vi "DidStop.vi"(6 "Wait for Module to stop?":bool, 7 "Exit via Stop Module Req?":bool, 8 "error in (no error)":errorcluster, 11 "ModuleAdmin":refnum<class "ModuleAdmin.lvclass">) -> (0 "error out":errorcluster, 3 "ModuleAdmin":refnum<class "ModuleAdmin.lvclass">)   [LabVIEW 2018, in "AcPwrPlugins.lvlib"]
doc: "This VI sends a stop message via a user event to Main.vi."
uses:
  AcPwrPlugins.lvlib
  <userlib>/NIST/ModuleAdminLib/ModuleAdmin/ModuleAdmin.lvclass
  AcPwrShared/clStopArgument.ctl
  AcPwrShared/clEventType.ctl
  AcPwrShared/AcPwrShared.lvlib
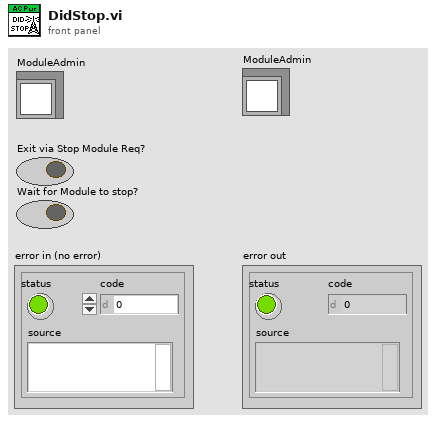
[diagram p1: front panel]
types:
  T1 = typedef "AcPwrShared.lvlib/clEventType.ctl" = cluster{"ModuleID":i32, "Data":variant}
  T2 = typedef "AcPwrShared.lvlib/clStopArgument.ctl" = cluster{"Exit via Stop Module Req?":bool, "Wait for Module to stop?":bool, "ModuleAdmin":refnum<class "ModuleAdmin.lvclass">}
  T3 = typedef "AcPwrShared.lvlib/clBroadcastEvents.ctl" = cluster{"DidInit":refnum<user-event>, "StatusUpdate":refnum<user-event>, "ErrorReport":refnum<user-event>, "DidStop":refnum<user-event>, "PathToINI":refnum<user-event>, "Measurements":refnum<user-event>, "LoadConfigFile":refnum<user-event>, "GetSettings":refnum<user-event>, "SetSettings":refnum<user-event>, "GetType&ID":refnum<user-event>, "GotSettings":refnum<user-event>}
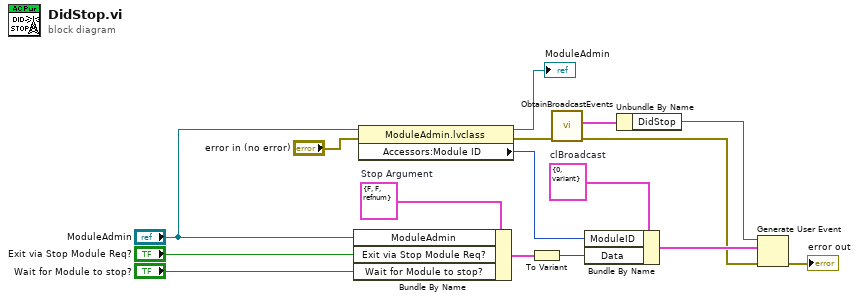
[diagram p0: block diagram]
diagram:
  w12 = T1 {"ModuleID"=0, "Data"=variant}  # clBroadcast
  w16 = T2 {"Exit via Stop Module Req?"=FALSE, "Wait for Module to stop?"=FALSE, "ModuleAdmin"=refnum}  # Stop Argument
  n1 = Bundle By Name(cluster=w16, "ModuleAdmin"="ModuleAdmin", "Exit via Stop Module Req?"="Exit via Stop Module Req?", "Wait for Module to stop?"="Wait for Module to stop?") -> (w14:T2)
  n2 = property class="ModuleAdmin.lvclass"(reference="ModuleAdmin", error in="error in (no error)") -> (reference out=→"ModuleAdmin":refnum<class "ModuleAdmin.lvclass">, error out=w2:errorcluster, "Accessors:Module ID"=w5:i32)
  n3 = To Variant(anything=w14) -> (Variant=w11:variant)
  n4 = call "ObtainBroadcastEvents.vi"("error in (no error)"=w2) -> ("error out"=w1:errorcluster, "clAcPwrEvents"=w15:T3)  [unwired: 9 in]
  n5 = Bundle By Name(cluster=w12, "ModuleID"=w5, "Data"=w11) -> (w10:T1)
  n6 = Unbundle By Name(w15) -> ("DidStop"=w13:refnum<user-event>)
  n7 = Generate User Event(user event=w13, event data cluster=w10, error in=w1) -> (error out=→"error out":errorcluster)  [unwired: 1 in, 1 out]
